vi "13.1 Propagate Data Types.vi"() -> ()   [LabVIEW 2019]
uses:
  13.1 Weather Data.ctl
  <vilib>/DAQmx/read.llb/DAQmx Read (Analog DBL 1Chan 1Samp).vi
  <vilib>/DAQmx/create/channels.llb/DAQmx Create Channel (AI-Temperature-Thermocouple).vi
  <vilib>/DAQmx/configure/timing.llb/DAQmx Timing (Sample Clock).vi
  <vilib>/DAQmx/miscellaneous.llb/DAQmx Fill In Error Info.vi
panel:
  in  "Lower Limit":dbl
  in  "Upper Limit":dbl
  out "Weather Data":T1
  in  "Stop":bool
  out "Waveform Chart":dbl(graph)
  in  "Configuration Cluster":T2={"Desired Sample Rate (Hz)"=-1.0, "sample mode"=10178, "Minimum value"=-1.0, "Maximum value"=-1.0, "Thermocouple Channel"="", "units"=10143, "thermocouple type"=10072} {"thermocouple type" items=["J"=10072, "K"=10073, "N"=10077, "R"=10082, "S"=10085, "T"=10086, "B"=10047, "E"=10055]; "units" items=["Deg C"=10143, "Deg F"=10144, "Kelvins"=10325, "Deg R"=10145, "From Custom Scale"=10065]; "sample mode" items=["Finite Samples"=10178, "Continuous Samples"=10123, "Hardware Timed Single Point"=12522]}
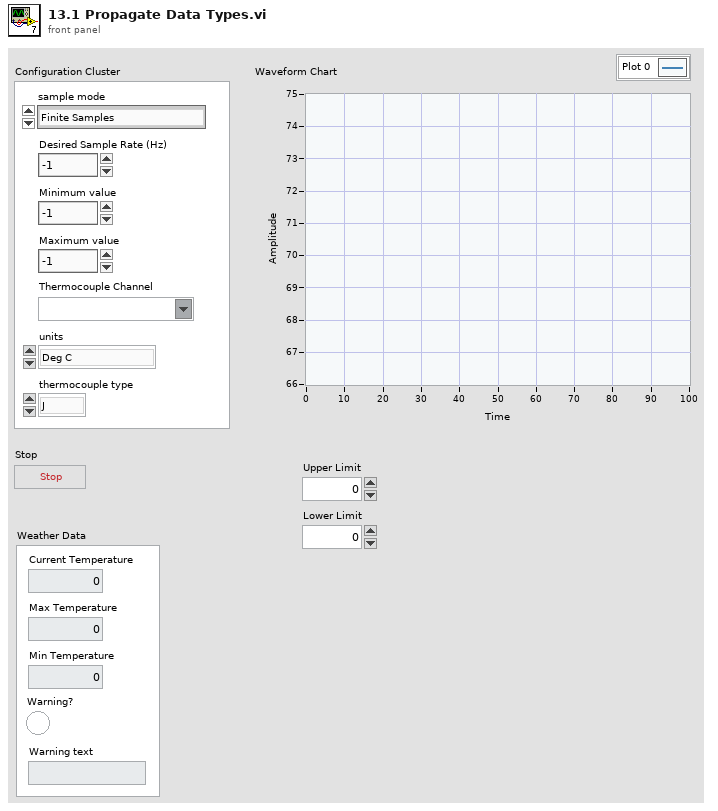
[diagram p1: front panel]
types:
  T1 = typedef "13.1 Weather Data.ctl" = cluster{"Current Temperature":dbl, "Max Temperature":dbl, "Min Temperature":dbl, "Warning?":bool, "Warning text":string}
  T2 = cluster{"Desired Sample Rate (Hz)":dbl, "sample mode":i32, "Minimum value":dbl, "Maximum value":dbl, "Thermocouple Channel":tag, "units":i32, "thermocouple type":i32}
  T3 = enum16{"open", "replace", "create", "open or create", "replace or create", "replace or create with confirmation"}
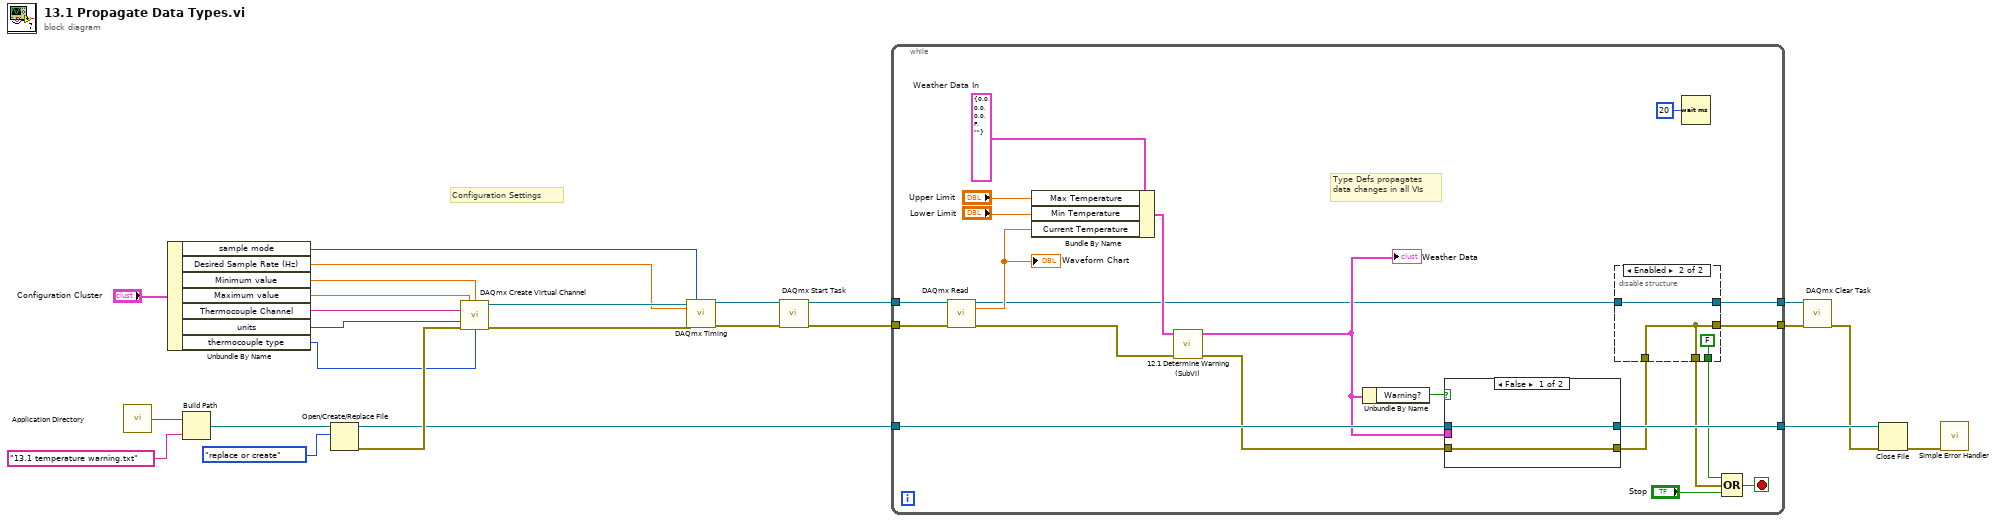
[diagram p0: block diagram]
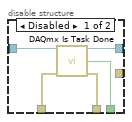
[diagram p2: hidden frame]
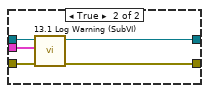
[diagram p3: hidden frame]
diagram:
  # "Configuration Settings"
  n1 = call <vilib>:"Application Directory.vi"() -> ("Application Directory"=w18:path)
  n2 = Unbundle By Name("Configuration Cluster") -> ("sample mode"=w13:i32, "Desired Sample Rate (Hz)"=w12:dbl, "Minimum value"=w11:dbl, "Maximum value"=w10:dbl, "Thermocouple Channel"=w9:tag, "units"=w8:i32, "thermocouple type"=w7:i32)
  n3 = Build Path(base path=w18, name or relative path="13.1 temperature warning.txt") -> (appended path=w20:path)
  n4 = Open/Create/Replace File(file path (use dialog)=w20, operation (0:open)=T3."replace or create") -> (refnum out=w6:refnum<file>, error out=w17:errorcluster)  [unwired: 4 in, 1 out]
  n5 = call-poly <vilib>:"DAQmx Create Virtual Channel.vi"("maximum value"=w10, "minimum value"=w11, "physical channels"=w9, "units"=w8, "error in"=w17, "thermocouple type"=w7) -> ("task out"=w24:refnum<k21>, "error out"=w23:errorcluster)  [unwired: 8 in]
  n6 = call-poly <vilib>:"DAQmx Timing.vi"("task/channels in"=w24, "sample mode"=w13, "rate"=w12, "error in"=w23) -> ("task out"=w21:refnum<k21>, "error out"=w22:errorcluster)  [unwired: 10 in]
  n7 = call <vilib>:"DAQmx Start Task.vi"("task/channels in"=w21, "error in"=w22) -> ("task out"=w15:refnum<k21>, "error out"=w16:errorcluster)  [unwired: 12 in]
  n8 = while {
    tunnel: w16 -> [w47]
    tunnel: w15 -> [w46]
    tunnel: w6 -> [w39]
    tunnel: [w31] -> w5
    tunnel: [w37] -> w4
    tunnel: [w26] -> w1
    stop <- w45 stop-if-true
    w36 = T1 {"Current Temperature"=0.0, "Max Temperature"=0.0, "Min Temperature"=0.0, "Warning?"=FALSE, "Warning text"=""}  # Weather Data In
    # "Type Defs propagates\ndata changes in all VIs"
    n9 = call-poly <vilib>:"DAQmx Read.vi"("task/channels in"=w46, "error in"=w47) -> ("task out"=w28:refnum<k21>, "data"=w41:dbl, "error out"=w40:errorcluster)  [unwired: 11 in]
    "Waveform Chart" <- w41
    n10 = Bundle By Name(cluster=w36, "Max Temperature"="Upper Limit", "Min Temperature"="Lower Limit", "Current Temperature"=w41) -> (w35:T1)
    n11 = call "12.1 Determine Warning (SubVI).vi"("Error In"=w40, "Weather Data In"=w35) -> ("Error Out"=w38:errorcluster, "Weather Data Out"=w34:T1)  [unwired: 8 in]
    "Weather Data" <- w34
    n12 = Unbundle By Name(w34) -> ("Warning?"=w33:bool)
    n13 = case shown="False" w33 {
      tunnel: w39 -> [w57 w62]
      tunnel: w38 -> [w56 w61]
      tunnel: [w56 w60] -> w30
      tunnel: [w57 w59] -> w37
      tunnel: w34 -> [_ w58]
      frame False {
      }
      frame True {
        n14 = call "13.1 Log Warning (SubVI).vi"("Error In"=w61, "Weather Data In"=w58, "refnum in"=w62) -> ("Error Out"=w60:errorcluster, "refnum out"=w59:refnum<file>)  [unwired: 7 in]
      }
    }
    n15 = disable-structure shown="Enabled" {
      disable-tunnel: [w52 w55] -> w31
      disable-tunnel: w30 -> [w51 w54]
      disable-tunnel: [w50 FALSE ("task done?")] -> w29
      disable-tunnel: w28 -> [w49 w55]
      disable-tunnel: [w48 w54] -> w27
      disable-tunnel: [_ w54] -> w26
      frame Disabled {
        n16 = call <vilib>:"DAQmx Is Task Done.vi"("task/channels in"=w49, "error in"=w51) -> ("task out"=w52:refnum<k21>, "task done?"=w50:bool, "error out"=w48:errorcluster)  [unwired: 11 in]
      }
      frame Enabled {
      }
    }
    n17 = Wait (ms)(milliseconds to wait=u32 20) -> ()  [unwired: 1 out]
    n18 = Compound Arithmetic op=OR(w29, w27, "Stop") -> (w45:bool)
  }
  n19 = call <vilib>:"DAQmx Clear Task.vi"("task in"=w5, "error in"=w1) -> ("error out"=w3:errorcluster)  [unwired: 13 in]
  n20 = Close File(refnum=w4, error in=w3) -> (error out=w2:errorcluster)  [unwired: 1 out]
  n21 = call <vilib>:"Simple Error Handler.vi"("error in (no error)"=w2) -> ()  [unwired: 4 in, 5 out]
